vi "SSL Tester with MQTT.vi"() -> ()   [LabVIEW 2016, in "AWS_IoT.lvlib"]
uses:
  AWS_IoT.lvlib
  MQTT/Controls/Connect_Flags.ctl
  MQTT/Controls/QoS.ctl
  MQTT/Controls/Will_Info.ctl
  MQTT/Controls/ConnectMeta.ctl
  MQTT/Controls/Retain_Flag.ctl
  MQTT/Controls/DUP_Flag.ctl
  Controls/certs.ctl
panel:
  in  "cert path":T1={"client cert file"=path "", "CA file"=path "", "client key file"=path ""}
  in  "Connect Meta":T2={"Retain"=TRUE, "DUP"=FALSE, "Keep Alive (sec)"=60, "QoS"=enum."At most once"}
  in  "MQTT Broker":cluster{"address (IP)":string, "port":u16}={"address (IP)"="youraddress.amazonaws.com", "port"=8883}
  in  "Will Info":T6={"Will message"="Last Will", "Will Topic"="Will Topic"}
  in  "Connect Flags":T7
  out "error out":errorcluster
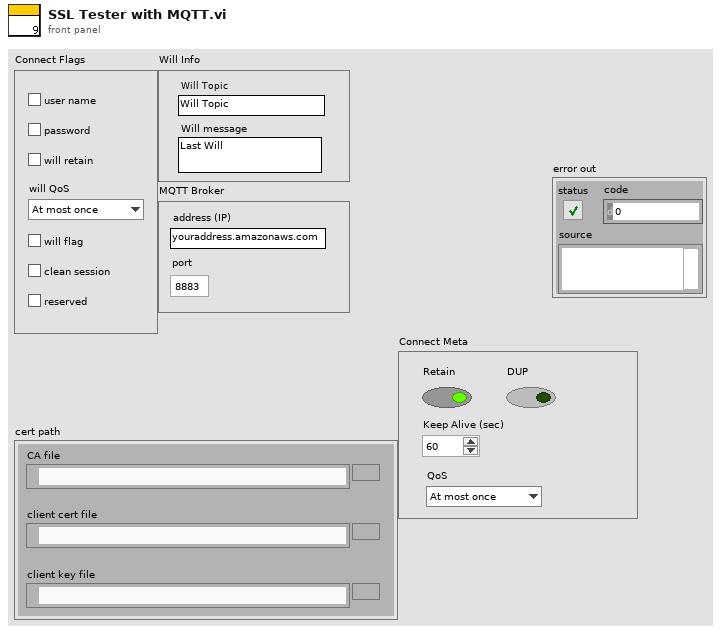
[diagram p1: front panel]
types:
  T1 = typedef "AWS_IoT.lvlib/certs.ctl" = cluster{"client cert file":path, "CA file":path, "client key file":path}
  T2 = typedef "ConnectMeta.ctl" = cluster{"Retain":T3, "DUP":T4, "Keep Alive (sec)":u16, "QoS":T5}
  T3 = typedef "Retain_Flag.ctl" = bool
  T4 = typedef "DUP_Flag.ctl" = bool
  T5 = typedef "QoS.ctl" = enum8{"At most once", "At least once", "Exactly once", "Reserved"}
  T6 = typedef "Will_Info.ctl" = cluster{"Will message":string, "Will Topic":string}
  T7 = typedef "Connect_Flags.ctl" = cluster{"user name":bool, "password":bool, "will retain":bool, "will flag":bool, "clean session":bool, "reserved":bool, "will QoS":T5}
  T8 = typedef "AWS_IoT.lvlib/SSL_Connection.ctl" = cluster{"connection ID":refnum<k5>, "TLS":cluster{"CXT ptr":i32, "SSL ptr":i32, "Socket ptr":i32}, "NIssleay library path":path, "server url":string}
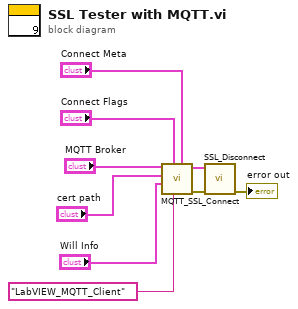
[diagram p0: block diagram]
diagram:
  n1 = call "MQTT_SSL_Connect.vi"("Connect Meta"="Connect Meta", "Client ID"="LabVIEW_MQTT_Client", "Connect Flags"="Connect Flags", "Will Info"="Will Info", "cert path"="cert path", "MQTT Broker"="MQTT Broker") -> ("error out"=w7:errorcluster, "SSL_Connection"=w8:T8)  [unwired: 3 in, 1 out]
  n2 = call "SSL_Disconnect.vi"("error in (no error)"=w7, "SSL_Connection"=w8) -> ("error out"=→"error out":errorcluster)  [unwired: 9 in]
